vi "ZZZ Chroma 1905x Series Example.vi"() -> ()   [LabVIEW 2025]
doc: "Contact Chroma\nTEL: +886-2-2298-3855 \nTEL: +886-3-397-5788 \nFAX: +886-2-2298-3596\nFAX: +886-3-327-4703 \nURL: http://www.chromaate.com \nE-mail: chroma@chroma.com.tw"
panel:
  in  "Reset":bool=TRUE
  in  "ID query":bool=TRUE
  out "ID":string
  out "System Error":string
  out "VISA session":refnum<visa-resource-name>
  in  "String":string="Chroma"
  out "error out":errorcluster
  in  "error in (no error)":errorcluster
  in  "STOP":bool
  in  "View Setups":bool
  in  "MEASURE":bool
  in  "SETUP":bool
  # "Initialization Control"
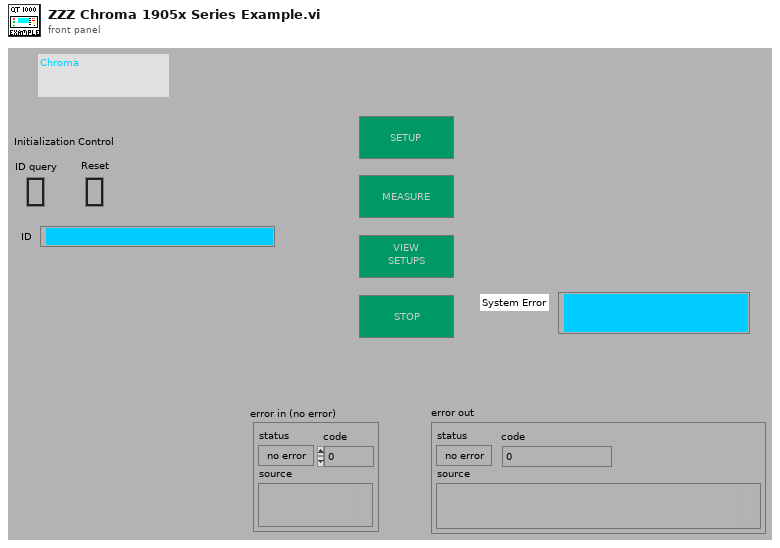
[diagram p1: front panel]
types:
  T1 = cluster{"error":bool, "code":i8, "source":string}
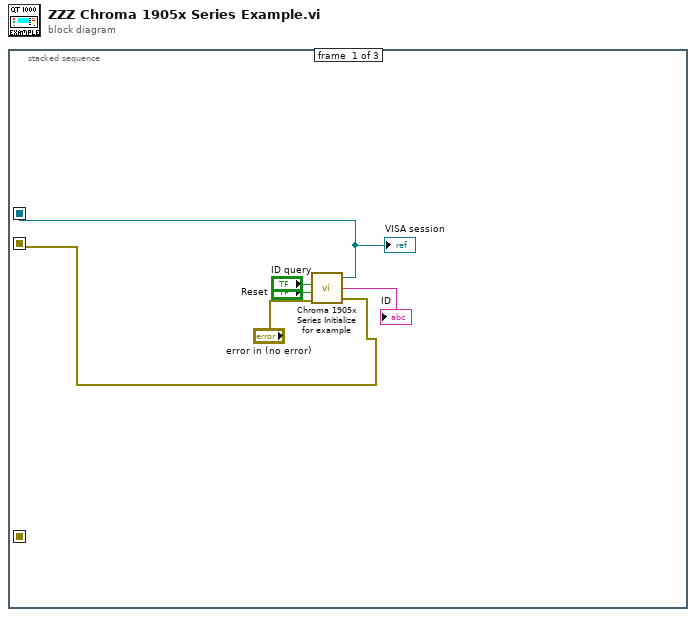
[diagram p0: block diagram]
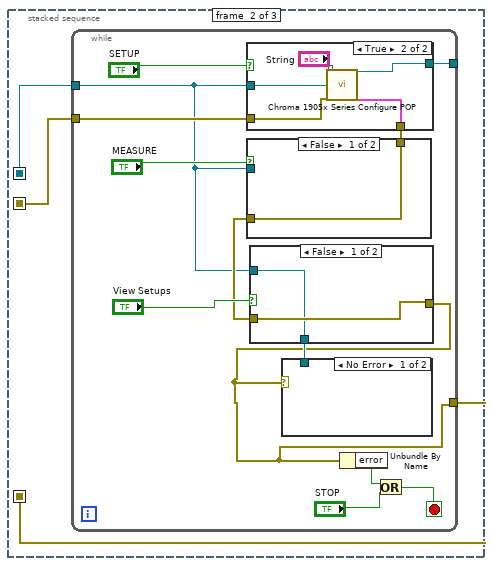
[diagram p2: hidden frame]
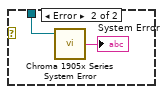
[diagram p3: hidden frame]
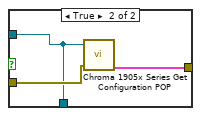
[diagram p4: hidden frame]
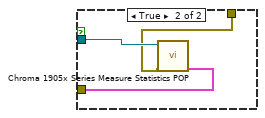
[diagram p5: hidden frame]
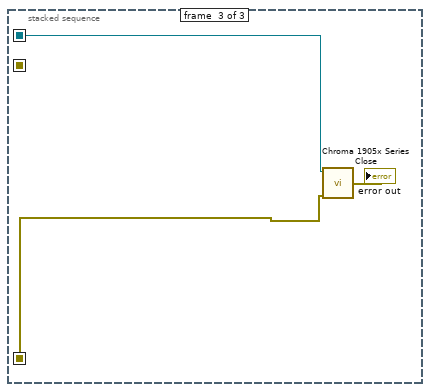
[diagram p7: hidden frame]
diagram:
  n1 = stacked-sequence {
    seq-local: [w3 _ _] -> [_ w9 w41]
    seq-local: [w6 _ _] -> [_ w8 _]
    seq-local: [_ w7 _] -> [_ _ w42]
    frame #0 {
      n2 = call "Chroma 1905x Series Initialize for example .vi"("error in (no error)"="error in (no error)", "reset"="Reset", "ID query"="ID query") -> ("error out"=w6:errorcluster, "Identification"=→"ID":string, "VISA session"=w3:refnum<visa-resource-name>)  [unwired: 1 in]
      "VISA session" <- w3
    }
    frame #1 {
      n3 = while {
        tunnel: [w10] -> w7
        tunnel: w8 -> [w18]
        tunnel: w9 -> [w15]
        tunnel: [w20] -> _
        stop <- w12 stop-if-true
        n4 = case shown="True" "SETUP" {
          tunnel: [w35 w39] -> w20
          tunnel: w15 -> [w35 w38]
          tunnel: w18 -> [w34 w37]
          tunnel: [w34 w36] -> w17
          frame False {
          }
          frame True {
            n5 = call "Chroma 1905x Series Configure POP.vi"("inst handle in"=w38, "error in"=w37) -> ("inst handle out"=w39:refnum<visa-resource-name>, "error out"=w36:T1)  [unwired: 23 in, 1 out]
          }
        }
        n6 = case shown="False" "MEASURE" {
          tunnel: w15 -> [_ w33]
          tunnel: w17 -> [w30 w32]
          tunnel: [w30 w31] -> w16
          frame False {
          }
          frame True {
            n7 = call "Chroma 1905x Series Measure Statistics POP.vi"("error in"=w32, "inst handle in"=w33) -> ("error out"=w31:T1)  [unwired: 2 in, 4 out]
          }
        }
        n8 = case shown="False" "View Setups" {
          tunnel: w15 -> [w25 w27]
          tunnel: w16 -> [w26 w29]
          tunnel: [w26 w28] -> w10
          tunnel: [w25 w27] -> w11
          frame False {
          }
          frame True {
            n9 = call "Chroma 1905x Series Get Configuration POP.vi"("inst handle in"=w27, "error in"=w29) -> ("error out"=w28:T1)  [unwired: 5 in, 1 out]
          }
        }
        n10 = case shown="No Error" w10 {
          tunnel: w11 -> [_ w24]
          frame No Error {
          }
          frame Error {
            n11 = call "Chroma 1905x Series System Error.vi"("inst handle in"=w24) -> ("System Error"=→"System Error":string)  [unwired: 2 in, 2 out]
          }
        }
        n12 = Unbundle By Name(w10) -> ("error"=w14:bool)
        n13 = Or(x=w14, y="STOP") -> (x .or. y?=w12:bool)
      }
    }
    frame #2 {
      n14 = call "Chroma 1905x Series Close.VI"("error in (no error)"=w42, "VISA session"=w41) -> ("error out"=→"error out":errorcluster)  [unwired: 2 in]
    }
  }
